vi "Run_Mnemonic_Command.vi"(6 "error in":errorcluster, 7 "command string":string, 8 "Device address":i32=4660 format="%x") -> (0 "error out":errorcluster, 2 "ACKS-array":u8[](array[numeric]) format="%x", 3 "ACKS count":i32, 4 "result count":i32, 5 "result-array":u8[](array[numeric]) format="%x")   [LabVIEW 2011]
doc: "Run Mnemonic Command - TI Version\n\n1. This VI is a simplification of the L-PSE VI. The L-PSE VI is called inside this VI. Only the key variables are available in this version of the VI. Some variables were intestinally omitted to simplify wiring. The original L-PSE version is available if you need access to all the variables (for more advanced operations). In the newest version of the shell, this VI also writes the command string, ACKS array, and result array to the string global variable which is used to populate the TI Debug VI.\na. Device address - USB-DAQ address.\nb. Command string - Mnemonic Command to USB DAQ (e.g. SPI CH1 BREH L 0x4A H).\nc. Error in - standard error input.\nd. Result count - the number of elements in the result array. Typically you will know how many results to expect based on the command you issue. However in some cases this output is useful. In most cases this output is not used.\ne. Result array - lists all the results for a given mnemonic command.\nf. ACKS Count - the number of elements in the ACKS array. Typically you will know how many ACKS to expect based on the command you issue. However in some cases this output is useful. In most cases this output is not used.\ng. ACKS Array - Used for acknowledge slave results on I2C communications. This is not used only for I2C commands and ignored for other commands.\nh. Error out - Errors will be issued for syntax errors, or hardware issues."
uses:
  INA231/Global Variables.vi
panel:
  out "Results Array":string[](array[string])
  out "ACKS Array":string[](array[string])
  out "Result Display":string
  out "ACKS Display":string
  out "Command String":string
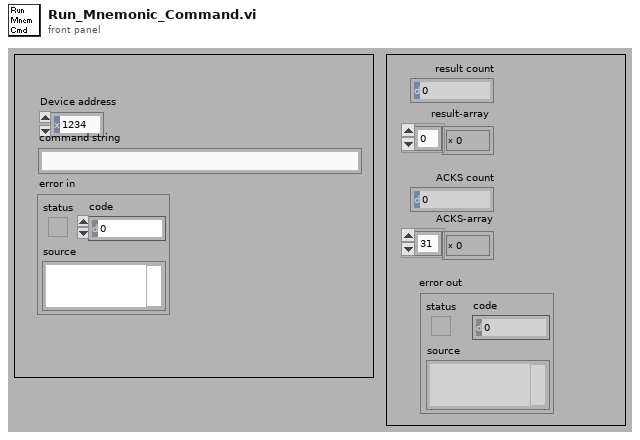
[diagram p1: front panel]
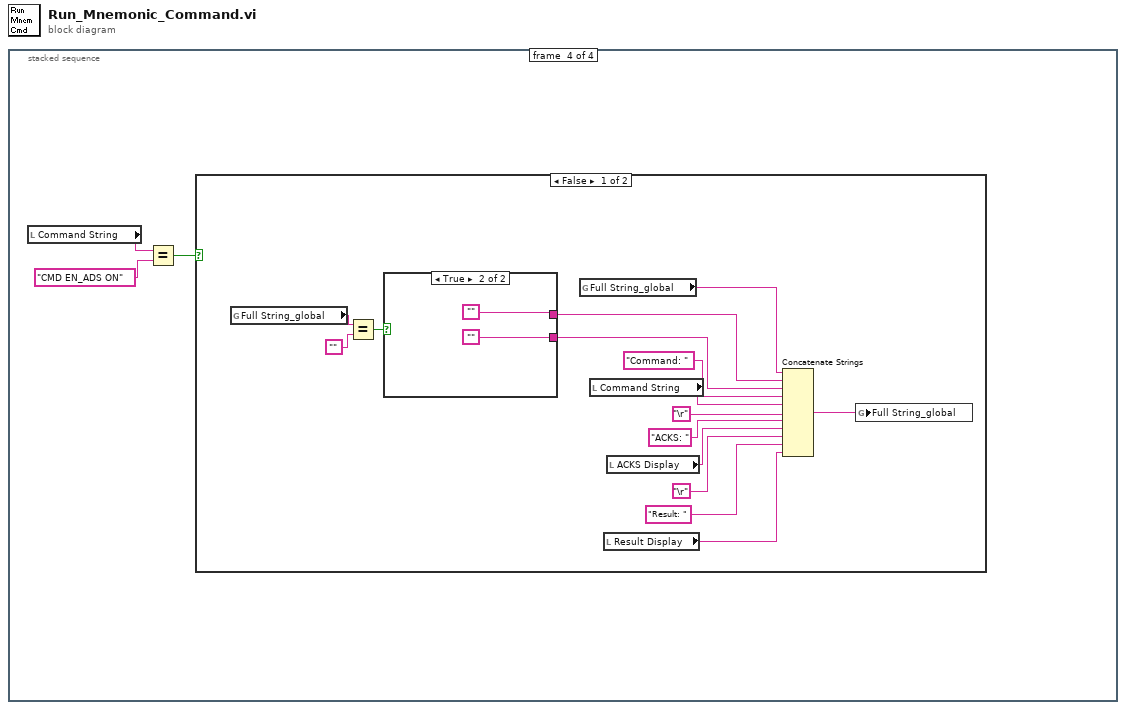
[diagram p0: block diagram]
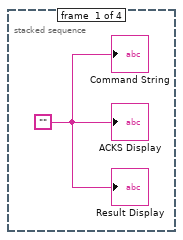
[diagram p2: hidden frame]
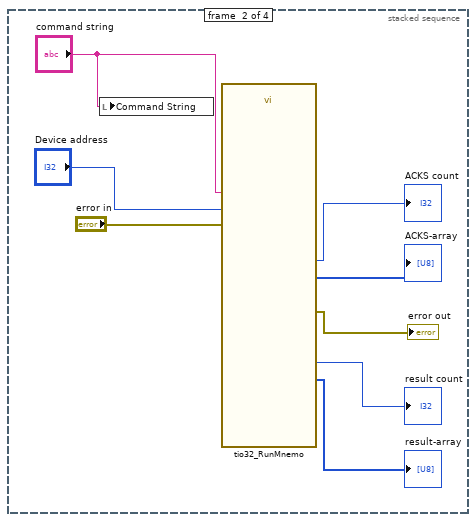
[diagram p3: hidden frame]
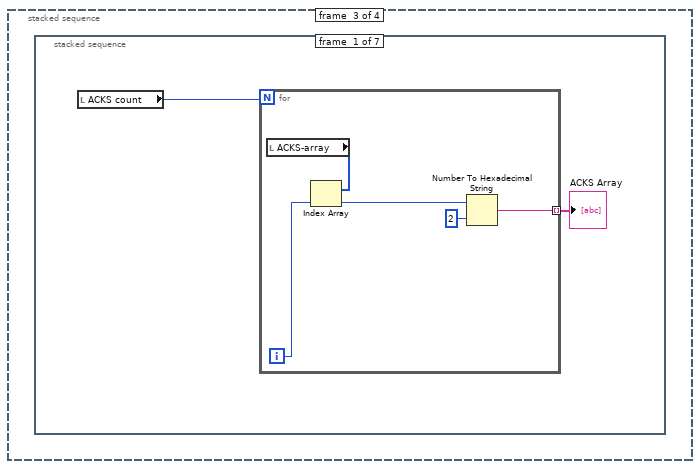
[diagram p4: hidden frame]
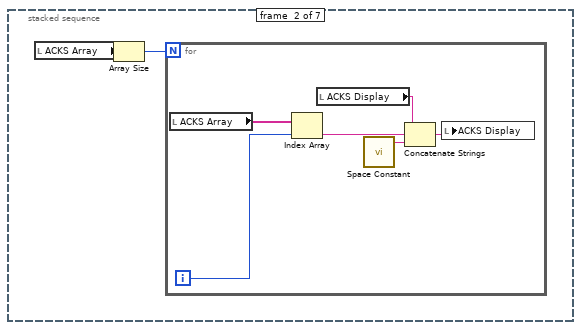
[diagram p5: hidden frame]
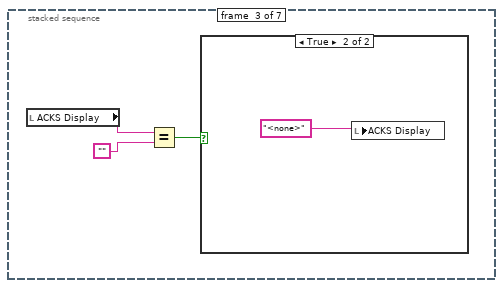
[diagram p6: hidden frame]
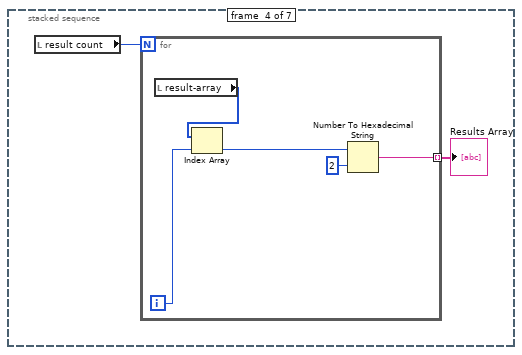
[diagram p8: hidden frame]
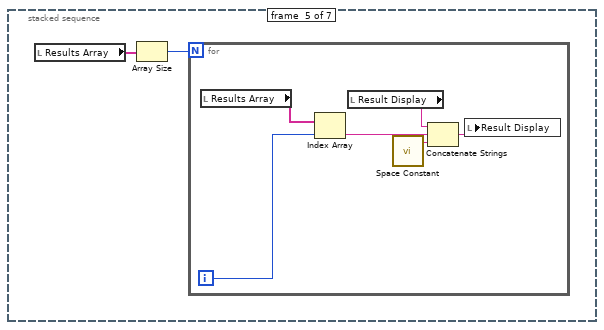
[diagram p9: hidden frame]
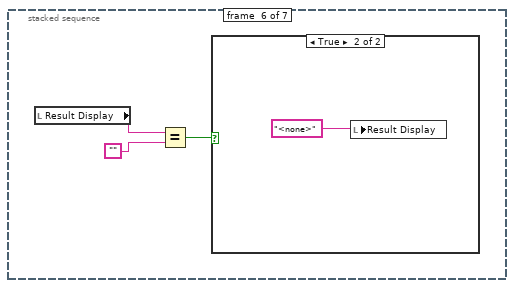
[diagram p10: hidden frame]
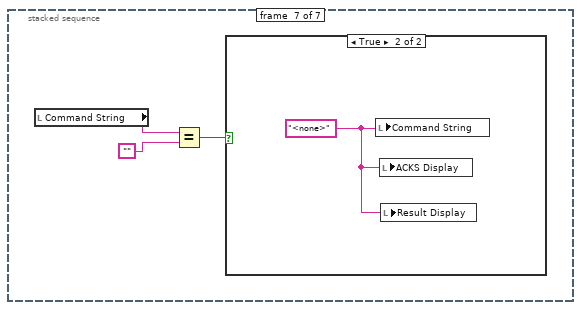
[diagram p12: hidden frame]
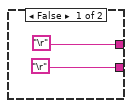
[diagram p14: hidden frame]
diagram:
  n1 = stacked-sequence {
    frame #0 {
      w1 = ""
      "Command String" <- w1
      "ACKS Display" <- w1
      "Result Display" <- w1
    }
    frame #1 {
      n2 = local write "Command String"("command string") -> ()
      n3 = call "tio32_RunMnemo.vi"("Device address"="Device address", "command string"="command string", "error in (no error)"="error in") -> ("result count"=→"result count":i32, "result-array"=→"result-array":u8[], "ACKS count"=→"ACKS count":i32, "ACKS-array"=→"ACKS-array":u8[], "error out"=→"error out":errorcluster)  [unwired: 6 in, 6 out]
    }
    frame #2 {
      n4 = stacked-sequence {
        frame #0 {
          n5 = local read "ACKS count"() -> (w11:i32)
          n6 = for {
            N: w11 -> [_]
            tunnel: [w13] -> w10 mode=indexing
            i -> [w16]
            n7 = local read "ACKS-array"() -> (w14:u8[])
            n8 = Index Array(array=w14, index=w16) -> (element=w15:u8)
            n9 = Number To Hexadecimal String(1:i16 2 ("width (-)"), 2:w15) -> (0:w13:string)
          }
          "ACKS Array" <- w10
        }
        frame #1 {
          n10 = local read "ACKS Array"() -> (w18:string[])
          n11 = Array Size(array=w18) -> (size(s)=w17:i32)
          n12 = for {
            N: w17 -> [_]
            i -> [w24]
            n13 = local read "ACKS Array"() -> (w23:string[])
            n14 = Index Array(array=w23, index=w24) -> (element=w20:string)
            n15 = local read "ACKS Display"() -> (w21:string)
            n16 = call <vilib>:"Space Constant.vi"() -> ("String"=w19:string)
            n17 = Concatenate Strings(w21, w20, w19) -> (w22:string)
            n18 = local write "ACKS Display"(w22) -> ()
          }
        }
        frame #2 {
          n19 = local read "ACKS Display"() -> (w25:string)
          n20 = Equal?(x=w25, y="") -> (x = y?=w27:bool)
          n21 = case shown="True" w27 {
            frame False {
            }
            frame True {
              n22 = local write "ACKS Display"("<none>") -> ()
            }
          }
        }
        frame #3 {
          n23 = local read "result count"() -> (w30:i32)
          n24 = for {
            N: w30 -> [_]
            tunnel: [w33] -> w29 mode=indexing
            i -> [w35]
            n25 = local read "result-array"() -> (w31:u8[])
            n26 = Index Array(array=w31, index=w35) -> (element=w34:u8)
            n27 = Number To Hexadecimal String(1:i16 2 ("width (-)"), 2:w34) -> (0:w33:string)
          }
          "Results Array" <- w29
        }
        frame #4 {
          n28 = local read "Results Array"() -> (w37:string[])
          n29 = Array Size(array=w37) -> (size(s)=w36:i32)
          n30 = for {
            N: w36 -> [_]
            i -> [w43]
            n31 = local read "Results Array"() -> (w41:string[])
            n32 = Index Array(array=w41, index=w43) -> (element=w42:string)
            n33 = local read "Result Display"() -> (w40:string)
            n34 = call <vilib>:"Space Constant.vi"() -> ("String"=w38:string)
            n35 = Concatenate Strings(w40, w42, w38) -> (w39:string)
            n36 = local write "Result Display"(w39) -> ()
          }
        }
        frame #5 {
          n37 = local read "Result Display"() -> (w44:string)
          n38 = Equal?(x=w44, y="") -> (x = y?=w46:bool)
          n39 = case shown="True" w46 {
            frame False {
            }
            frame True {
              n40 = local write "Result Display"("<none>") -> ()
            }
          }
        }
        frame #6 {
          n41 = local read "Command String"() -> (w48:string)
          n42 = Equal?(x=w48, y="") -> (x = y?=w50:bool)
          n43 = case shown="True" w50 {
            frame False {
            }
            frame True {
              w51 = "<none>"
              n44 = local write "Command String"(w51) -> ()
              n45 = local write "ACKS Display"(w51) -> ()
              n46 = local write "Result Display"(w51) -> ()
            }
          }
        }
      }
    }
    frame #3 {
      n47 = local read "Command String"() -> (w52:string)
      n48 = Equal?(x=w52, y="CMD EN_ADS ON") -> (x = y?=w53:bool)
      n49 = case shown="False" w53 {
        frame False {
          n50 = global read "Global Variables.vi" "Full String_global"() -> (w66:string)
          n51 = Equal?(x=w66, y="") -> (x = y?=w65:bool)
          n52 = case shown="True" w65 {
            tunnel: ["\r" ""] -> w68
            tunnel: ["\r" ""] -> w69
            frame False {
            }
            frame True {
            }
          }
          n53 = global read "Global Variables.vi" "Full String_global"() -> (w56:string)
          n54 = local read "Command String"() -> (w58:string)
          n55 = local read "Result Display"() -> (w64:string)
          n56 = local read "ACKS Display"() -> (w61:string)
          n57 = Concatenate Strings(w56, w68, w69, "Command: ", w58, "\r", "ACKS: ", w61, "\r", "Result: ", w64) -> (w55:string)
          n58 = global write "Global Variables.vi" "Full String_global"(w55) -> ()
        }
        frame True {
        }
      }
    }
  }
